vi "Wait Scan2.vi"(8 "error in (no error)":errorcluster, 9 "Clust Refnum":refnum<vi>, 10 "number":u32, 11 "Data In":T2) -> (0 "error out":errorcluster, 1 "States":T1=enum."Initialize", 3 "Data Out":T2)   [LabVIEW 2014]
doc: "Use this template to build a standard state machine design pattern. Each state executes code and determines which state to transition to. Contrast this design pattern with the User Interface Event Handler pattern, in which code executes in response to user actions. Contrast this design pattern also with the Queued Message Handler pattern, in which each message handling code can queue zero or more new messages.\nNote: This template does not contain the most recent programming guidelines recommended by National Instruments. For a complete, project-based implementation of the Standard State Machine pattern, use the Create Project dialog box instead of this template."
uses:
  controls/Data1.ctl
  controls/Payjson.ctl
  controls/State.ctl
  controls/Wait Scan States.ctl
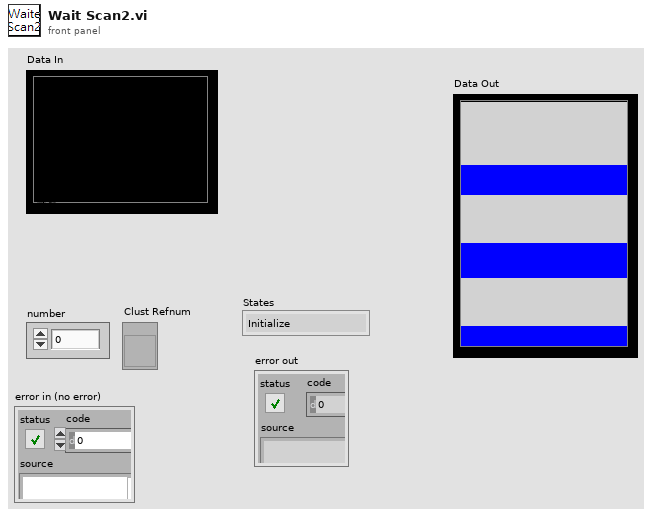
[diagram p1: front panel]
types:
  T1 = typedef "State.ctl" = enum16{"int", "Initalize0", "Initialize", "Wait for Scan", "State 1", "State 2", "NG", "NG1", "OK", "OKNG", "OKNG1", "Exit"}
  T2 = typedef "Data1.ctl" = cluster{"Date":string, "BarCode1":string, "BarCode2":string, "BarCode3":string, "Message":string, "OK Count":u16, "NG Count":u16, "Total Count":u16, "ModelData":string[][], "OK&NG":bool, "COM1":refnum<visa-resource-name>, "COM2":refnum<visa-resource-name>, "IO":i32, "Time":u32, "TCP":refnum<k5>, "TCP 2":refnum<k5>, "COM1 2":refnum<visa-resource-name>, "CheckNum":string, "BarCode1_1":string, "BarCode2_1":string, "BarCode3_1":string, "日期":string, "機種":string, "機號":string, "商品條碼1":string, "OK_1":string, "OK":string, "NG":string, "NG_1":string, "Total":string, "Total_1":string, "ClaerTime":u32, "Pjson":T3, "LotNo":string[], "CheckParsArray":string[], "BarCode4":string, "BarCode4_1":string, "商品條碼2":string, "BarCode5":string, "BarCode5_1":string, "商品條碼3":string, "ReScanNG":i32, "NGTimeCT":u32}
  T3 = typedef "Payjson.ctl" = cluster{"DEPT":string, "LINE":string, "STANO":string, "WORKNO":string, "PRODSN":string, "COMPNTID":string, "COMPNTLOT":string, "COMPNTSN":string, "USEDQTY":i16, "OPDATE":string, "OPUSER":string, "RECVDATE":string, "MMODU":string}[]
  T4 = typedef "Wait Scan States.ctl" = enum16{"Initialize", "State1", "Stop"}
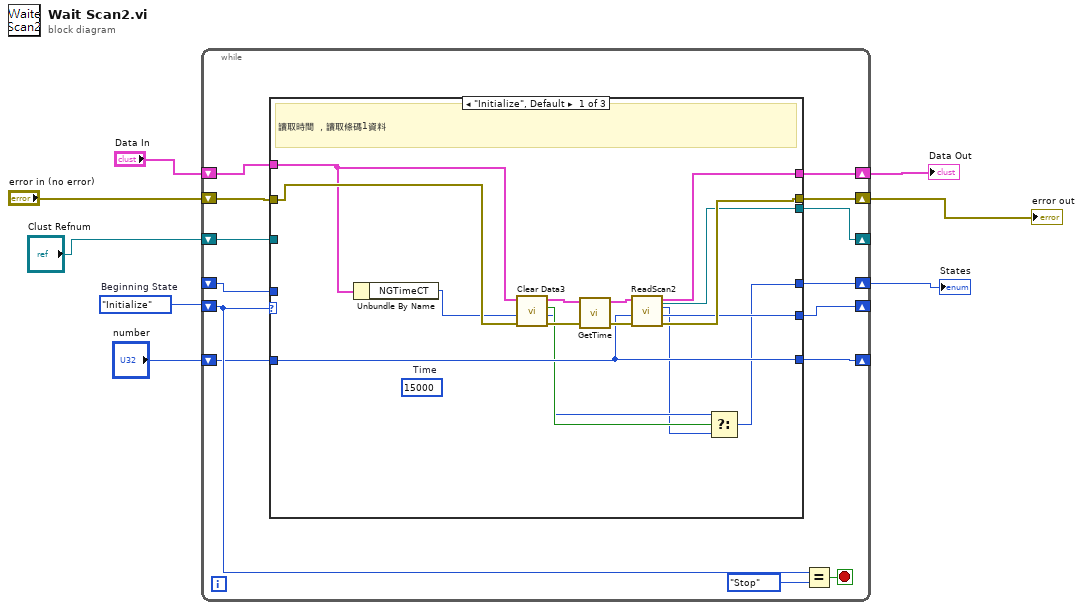
[diagram p0: block diagram]
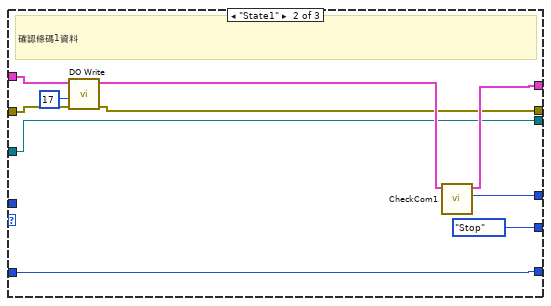
[diagram p2: hidden frame]
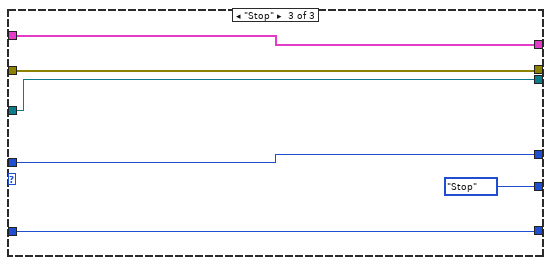
[diagram p3: hidden frame]
diagram:
  w8 = Wait_Scan_States."Initialize"  # Beginning State
  n1 = while {
    shift-right: [w19] -> _
    shift-left: w8 -> [w20]
    shift-right: [w16] -> w6
    shift-left: "Data In" -> [w18]
    shift-right: [w15] -> w3
    shift-left: "error in (no error)" -> [w17]
    shift-right: [w14] -> w4
    shift-left: _ -> [w13]
    shift-right: [w12] -> _
    shift-left: "Clust Refnum" -> [w11]
    shift-right: [w9] -> _
    shift-left: "number" -> [w10]
    stop <- w22 stop-if-true
    n2 = case shown="\"Initialize\", Default" w20 {
      tunnel: [w31 Wait_Scan_States."Stop" ("Next State") Wait_Scan_States."Stop" ("Next State")] -> w19
      tunnel: w18 -> [w28 w44 w51]
      tunnel: w17 -> [w33 w42 w50]
      tunnel: [w35 w46 w51] -> w16
      tunnel: [w36 w39 w50] -> w15
      tunnel: [w23 w45 w52] -> w14
      tunnel: w13 -> [_ _ w52]
      tunnel: [w29 w38 w49] -> w12
      tunnel: w11 -> [_ w38 w49]
      tunnel: w10 -> [w30 w41 w48]
      tunnel: [w30 w41 w48] -> w9
      frame "Initialize", Default {
        (unwired) u32 15000  # Time
        # "讀取時間 ，讀取條碼1資料"
        n3 = Unbundle By Name(w28) -> ("NGTimeCT"=w27:u32)
        n4 = call "Clear Data3.vi"("Data In"=w28, "Time"=w27, "error in (no error)"=w33) -> ("Data Out"=w34:T2, "Timeout"=w26:bool, "State"=w25:T1, "error out"=w32:errorcluster)  [unwired: 4 in]
        n5 = call "GetTime.vi"("Data In"=w34) -> ("Data Out"=w37:T2)  [unwired: 10 in]
        n6 = call "ReadScan2.vi"("error in (no error)"=w32, "number"=w30, "Data In"=w37) -> ("error out"=w36:errorcluster, "Next State"=w31:T4, "States"=w24:T1, 3:"Data Out"=w35:T2, 5:"Data Out"=w29:refnum<vi>)  [unwired: 4 in]
        n7 = Select(t=w25, s=w26, f=w24) -> (s? t:f=w23:T1)
      }
      frame "State1" {
        # "確認條碼1資料"
        n8 = call "DO Write.vi"("error in (no error)"=w42, "data"=u8 17, "Data In"=w44) -> ("error out"=w39:errorcluster, "Data Out"=w43:T2)  [unwired: 7 in]
        n9 = call "CheckCom1.vi"("Data In"=w43) -> ("States"=w45:T1, "Data Out"=w46:T2)  [unwired: 9 in]
      }
      frame "Stop" {
      }
    }
    n10 = Equal?(x=w20, y=Wait_Scan_States."Stop" ("States")) -> (x = y?=w22:bool)
  }
  "Data Out" <- w6
  "error out" <- w3
  "States" <- w4
